vi "AlliGator Export Single Phasor Plot Phase Lifetimes.vi"(6 "Frequency":dbl[unit], 8 "Error In":errorcluster, 9 "File Path in (empty: dialog)":path, 10 "Plot Idx (-1: last)":i32=-1, 11 "Phasor Graph":refnum<vi>) -> (0 "Error Out":errorcluster, 1 "File Path out":path, 2 "Message":string)   [LabVIEW 2021, in "AlliGator Phasor Graph.lvlib"]
doc: "Saves phase lifetime for the selected phasor plot to an ASCII file."
uses:
  AlliGator Phasor Graph.lvlib
  0c687634-756e-4512-a17a-756a9e49c85b.vi
  <vilib>/Utility/file.llb/Write Delimited Spreadsheet (DBL).vi
  Graphs/XY Graph/XY Graph Add-Ons.lvlib
  Arrays/Arrays.lvlib
  <vilib>/Analysis/NI_AALBase.lvlib
  Phasor/Phasor.lvlib
panel:
  # "see the AlliGator License on the block diagram (Ctrl+E or Window:Show Block Diagram)"
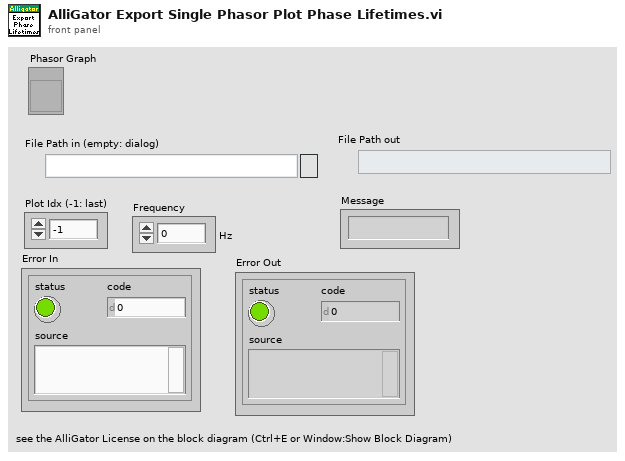
[diagram p1: front panel]
types:
  T1 = cluster{"Numeric Control":dbl, "Numeric Control":dbl}[]
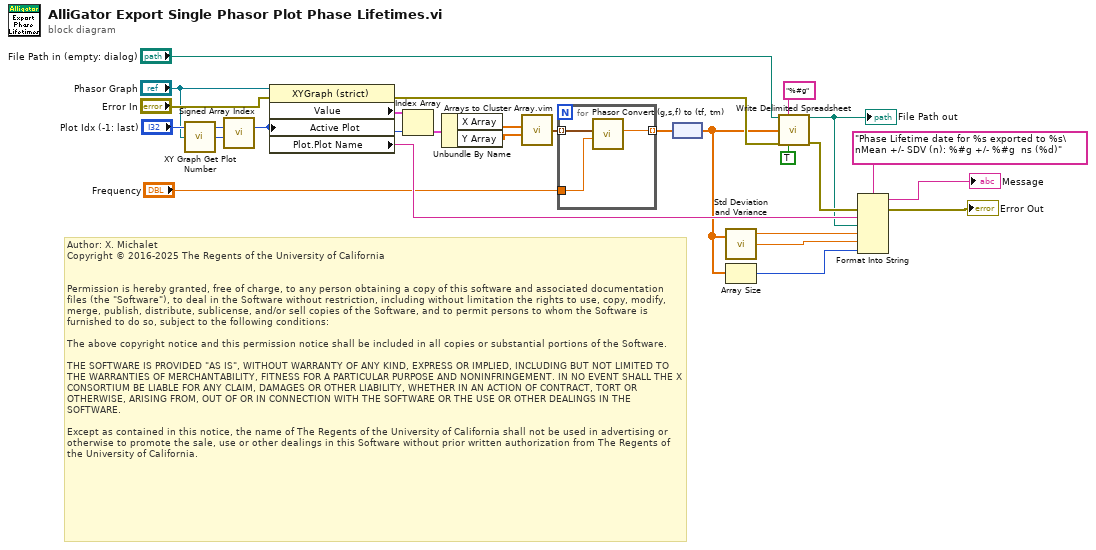
[diagram p0: block diagram]
diagram:
  # "Author: X. Michalet\nCopyright © 2016-2025 The Regents of the University of California\n \n\nPermission is hereby granted, free of charge, to any person obtaining a copy of this software and associated documentation files (the \"Software\"), to deal in the Software without restriction, including without limitation the rights to use, copy, modify, merge, publish, distribute, sublicense, and/or sell copies of the Software, and to permit persons to whom the Software is furnished to do so, subject to the following conditions:\n\nThe above copyright notice and this permission notice shall be included in all copies or substantial portions of the Software.\n\nTHE SOFTWARE IS PROVIDED \"AS IS\", WITHOUT WARRANTY OF ANY KIND, EXPRESS OR IMPLIED, INCLUDING BUT NOT LIMITED TO THE WARRANTIES OF MERCHANTABILITY, FITNESS FOR A PARTICULAR PURPOSE AND NONINFRINGEMENT. IN NO EVENT SHALL THE X CONSORTIUM BE LIABLE FOR ANY CLAIM, DAMAGES OR OTHER LIABILITY, WHETHER IN AN ACTION OF CONTRACT, TORT OR OTHERWISE, ARISING FROM, OUT OF OR IN CONNECTION WITH THE SOFTWARE OR THE USE OR OTHER DEALINGS IN THE SOFTWARE.\n\nExcept as contained in this notice, the name of The Regents of the University of California shall not be used in advertising or otherwise to promote the sale, use or other dealings in this Software without prior written authorization from The Regents of the University of California."
  n1 = call "XY Graph Get Plot Number.vi"("XYGraph"="Phasor Graph") -> ("# Plots"=w24:i32)  [unwired: 8 in]
  n2 = call "Signed Array Index.vi"("Array Size"=w24, "Array Index in"="Plot Idx (-1: last)") -> ("Array Index out"=w22:i32)  [unwired: 9 in]
  n3 = property class="XYGraph (strict)"(reference="Phasor Graph", error in="Error In", "Active Plot"=w22) -> (error out=w18:errorcluster, "Value"=w25:cluster{"X Array":dbl[], "Y Array":dbl[]}[], "Plot.Plot Name"=w15:string)  [unwired: 1 out]
  n4 = Index Array(array=w25, index=w22) -> (element=w7:cluster{"X Array":dbl[], "Y Array":dbl[]})
  n5 = Unbundle By Name(w7) -> ("X Array"=w6:dbl[], "Y Array"=w5:dbl[])
  n6 = call "Arrays to Cluster Array.vim"("Array 1"=w6, "Array 2"=w5) -> ("Cluster Array"=w4:T1)  [unwired: 6 in]
  n7 = for {
    tunnel: w4 -> [w29] mode=indexing
    tunnel: "Frequency" -> [w28]
    tunnel: [w27] -> w2 mode=indexing
    n8 = call "Phasor Convert (g,s,f) to (tf, tm).vi"("Phasor Harmonic Frequency"=w28, "Phasor (g, s)"=w29) -> ("Phase Lifetime"=w27:dbl[unit])  [unwired: 7 in, 2 out]
  }
  n9 = node(w2) -> (w1:dbl[])
  n10 = call <vilib>:"Std Deviation and Variance.vi"("X"=w1) -> ("mean"=w14:dbl, "standard deviation"=w13:dbl)  [unwired: 1 in, 1 out]
  n11 = Array Size(array=w1) -> (size(s)=w10:i32)
  n12 = call-poly <vilib>:"Write Delimited Spreadsheet.vi"("file path (dialog if empty)"="File Path in (empty: dialog)", "format (%.3f)"="%#g", "1D data"=w1, "error in (no error)"=w18, "transpose? (no:F)"=TRUE) -> ("new file path (Not A Path if cancelled)"=w11:path, "error out"=w12:errorcluster)  [unwired: 9 in]
  "File Path out" <- w11
  n13 = Format Into String(format string="Phase Lifetime date for %s exported to %s\nMean +/- SDV (n): %#g +/- %#g  ns (%d)", error in=w12, w15, w11, w14, w13, w10) -> (resulting string=→"Message":string, error out=→"Error Out":errorcluster)  [unwired: 1 in]
